vi "Get Top Scores.vi"(10 "Challenge":refnum<class "Challenge.lvclass">, 11 "SQLite":refnum<class "SQLite.lvclass">) -> (0 "error out":errorcluster, 3 "Top Scores":T1[](array[typedef]))   [LabVIEW 2020, in "Summer of LabVIEW.lvlib" / "Challenges.lvclass"]
uses:
  Challenges.lvclass
  SQLite/SQLite.lvclass
  User Score.ctl
  SoL Scoring/Score.ctl
  SoL Scoring/Score Entry.ctl
  Challenge/Challenge.lvclass
  <vilib>/drjdpowell/SQLite Library/SQL Statement/SQL Statement.lvclass/SQL Statement.ctl
  <vilib>/drjdpowell/SQLite Library/SQL Statement/Column I64.vi
  <vilib>/drjdpowell/SQLite Library/SQL Statement/Bind Integer.vi
  <vilib>/drjdpowell/SQLite Library/SQL Statement/Error Message.vi
  <vilib>/drjdpowell/SQLite Library/SQL Statement/Column String.vi
  Challenges.lvclass/Challenges.ctl
  <vilib>/drjdpowell/SQLite Library/SQL Connection/Connection.lvclass
  <vilib>/drjdpowell/SQLite Library/SQL Statement/SQL Statement.lvclass
  SoL Scoring/SoL Scoring.lvlib
  Summer of LabVIEW.lvlib
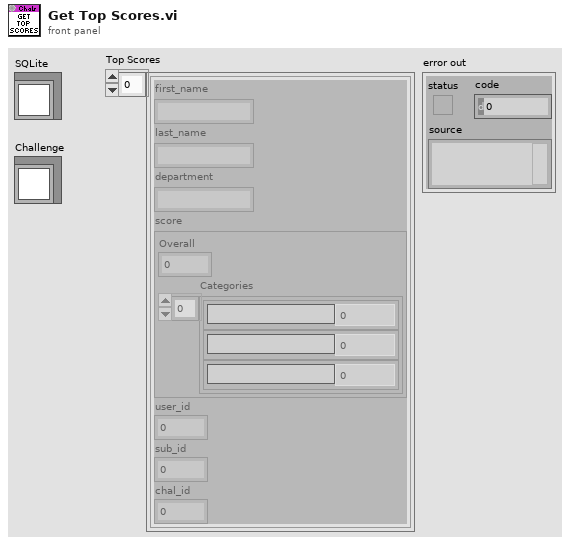
[diagram p1: front panel]
types:
  T1 = typedef "Summer of LabVIEW.lvlib/User Score.ctl" = cluster{"first_name":string, "last_name":string, "department":string, "score":T2, "user_id":i64, "sub_id":i64, "chal_id":i64}
  T2 = typedef "SoL Scoring.lvlib/Score.ctl" = cluster{"Overall":dbl, "Categories":T3[]}
  T3 = typedef "SoL Scoring.lvlib/Score Entry.ctl" = cluster{"Category":string, "Value":dbl}
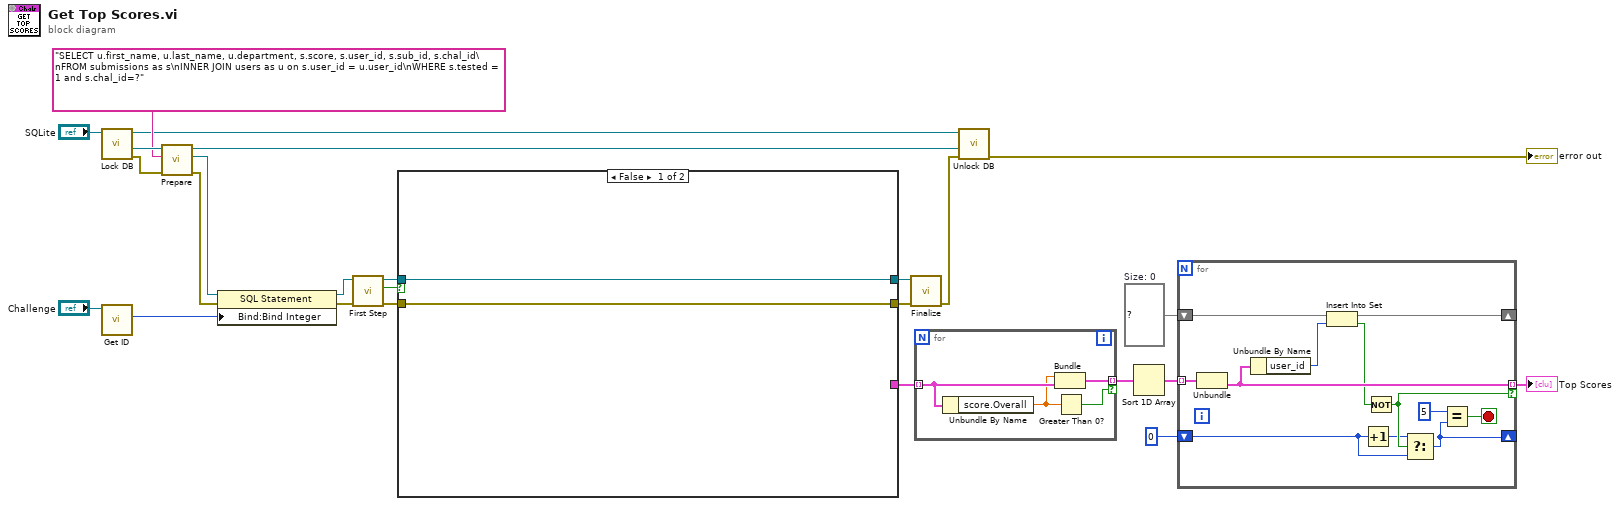
[diagram p0: block diagram]
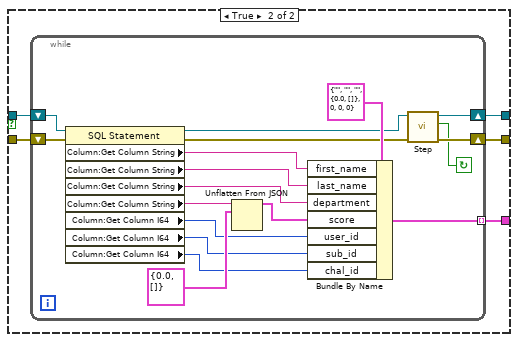
[diagram p2: hidden frame]
diagram:
  w2 = set{i64} {}  # Size: 0
  n1 = call "Lock DB.vi"("SQLite in"="SQLite") -> ("error out"=w19:errorcluster, "SQLite DB"=w24:refnum<class "Connection.lvclass">, "SQLite out"=w10:refnum<class "SQLite.lvclass">)  [unwired: 7 in, 1 out]
  n2 = call "Get ID.vi"("Challenge in"="Challenge") -> ("ID"=w20:i64)  [unwired: 9 in, 1 out]
  n3 = call <vilib>:"Prepare.vi"("error in (no error)"=w19, "SQL"="SELECT u.first_name, u.last_name, u.department, s.score, s.user_id, s.sub_id, s.chal_id\nFROM submissions as s\nINNER JOIN users as u on s.user_id = u.user_id\nWHERE s.tested = 1 and s.chal_id=?", "SQLite Connection in"=w24) -> ("error out"=w18:errorcluster, "SQL Statement"=w22:refnum<class "SQL Statement.lvclass">, "SQLite Connection"=w8:refnum<class "Connection.lvclass">)  [unwired: 4 in, 2 out]
  n4 = property class="SQL Statement"(reference=w22, error in=w18, "Bind:Bind Integer"=w20) -> (reference out=w17:refnum<class "SQL Statement.lvclass">, error out=w16:errorcluster)
  n5 = call <vilib>:"First Step.vi"("error in (no error)"=w16, "SQL Statement in"=w17) -> ("error out"=w13:errorcluster, "Row returned"=w15:bool, "SQL Statement"=w14:refnum<class "SQL Statement.lvclass">)  [unwired: 7 in]
  n6 = case shown="False" w15 {
    tunnel: w14 -> [w27 w32]
    tunnel: w13 -> [w26 w31]
    tunnel: [w27 w30] -> w11
    tunnel: [w26 w29] -> w12
    tunnel: [_ w28] -> w7
    frame False {
    }
    frame True {
      n7 = while {
        shift-right: [w35] -> w30
        shift-left: w32 -> [w50]
        tunnel: [w38] -> w28 mode=indexing
        shift-right: [w34] -> w29
        shift-left: w31 -> [w49]
        stop <- w33 continue-if-true
        n8 = property class="SQL Statement"(reference=w50, error in=w49) -> (reference out=w36:refnum<class "SQL Statement.lvclass">, error out=w37:errorcluster, "Column:Get Column String"=w47:string, "Column:Get Column String"=w46:string, "Column:Get Column String"=w45:string, "Column:Get Column String"=w44:string, "Column:Get Column I64"=w41:i64, "Column:Get Column I64"=w40:i64, "Column:Get Column I64"=w39:i64)
        n9 = Unflatten From JSON(JSON string=w44, type and defaults=T2 {"Overall"=0.0, "Categories"=[]} ("Score")) -> (value=w42:T2)  [unwired: 5 in, 1 out]
        n10 = Bundle By Name(cluster=T1 {"first_name"="", "last_name"="", "department"="", "score"={"Overall"=0.0, "Categories"=[]}, "user_id"=0, "sub_id"=0, "chal_id"=0} ("User Score"), "first_name"=w47, "last_name"=w46, "department"=w45, "score"=w42, "user_id"=w41, "sub_id"=w40, "chal_id"=w39) -> (w38:T1)
        n11 = call <vilib>:"Step.vi"("error in (no error)"=w37, "SQL Statement in"=w36) -> ("error out"=w34:errorcluster, "Row returned"=w33:bool, "SQL Statement"=w35:refnum<class "SQL Statement.lvclass">)  [unwired: 7 in]
      }
    }
  }
  n12 = call <vilib>:"Finalize.vi"("error in (no error)"=w12, "SQL Statement in"=w11) -> ("error out"=w9:errorcluster)  [unwired: 9 in]
  n13 = for {
    tunnel: w7 -> [w54] mode=indexing
    tunnel: [w53] -> w6 mode=indexing if=w51
    n14 = Unbundle By Name(w54) -> ("score.Overall"=w52:dbl)
    n15 = Bundle("Overall"=w52, "User Score"=w54) -> (w53:cluster{"Overall":dbl, "User Score":T1})  [unwired: 1 in]
    n16 = Greater Than 0?(x=w52) -> (x > 0?=w51:bool)
  }
  n17 = call "Unlock DB.vi"("error in (no error)"=w9, "SQLite DB"=w8, "SQLite in"=w10) -> ("error out"=→"error out":errorcluster)  [unwired: 7 in, 1 out]
  n18 = Sort 1D Array(array=w6) -> (sorted array=w3:cluster{"Overall":dbl, "User Score":T1}[])
  n19 = for {
    tunnel: w3 -> [w66] mode=indexing
    tunnel: [w65] -> w5 mode=indexing if=w60
    shift-right: [w61] -> _
    shift-left: w2 -> [w64]
    shift-right: [w57] -> _
    shift-left: 0 -> [w58]
    stop <- w55 stop-if-true
    n20 = Unbundle(w66) -> ("User Score"=w65:T1)  [unwired: 1 out]
    n21 = Unbundle By Name(w65) -> ("user_id"=w63:i64)
    n22 = Insert Into Set(10:w63, 11:w64) -> (2:w62:bool, 3:w61:set{i64})
    n23 = Increment(x=w58) -> (x+1=w59:i32)
    n24 = Not(x=w62) -> (.not. x?=w60:bool)
    n25 = Select(t=w59, s=w60, f=w58) -> (s? t:f=w57:i32)
    n26 = Equal?(x=5, y=w57) -> (x = y?=w55:bool)
  }
  "Top Scores" <- w5
